vi "data analysis5.vi"() -> ()   [LabVIEW 2022 SP3]
uses:
  <vilib>/Utility/file.llb/Read From Spreadsheet File (DBL).vi
  <vilib>/Utility/file.llb/Read From Spreadsheet File (string).vi
  <vilib>/Utility/file.llb/Write To Spreadsheet File (DBL).vi
  <vilib>/Analysis/NI_AALBase.lvlib
panel:
  out "x+y 2":i32
  out "String converted to Time Stamp 2":timestamp
  out "output 2":timestamp
  out "Array":timestamp[](array[timestamp])
  out "Cursor.Cursor Position:Cursor X":dbl
  in  "Ring":u16(ring) items=["Temperature", "Humidity"]
  out "x+y":i32
  out "String converted to Time Stamp":timestamp
  out "Raw Data":dbl[][](graph)
  out "Time":string[](array[string])
  out "Temp":dbl[](array[numeric])
  out "Humid":dbl[](array[numeric])
  out "Current Data":dbl[](graph)
  in  "Log data value":bool
  out "standard deviation":dbl format="%0.2f"
  out "mean":dbl format="%0.2f"
  in  "stop":bool
  out "Data Section":dbl[][](graph)
  in  "Path":path=path "C:/Users/Deely/Desktop/test.txt"
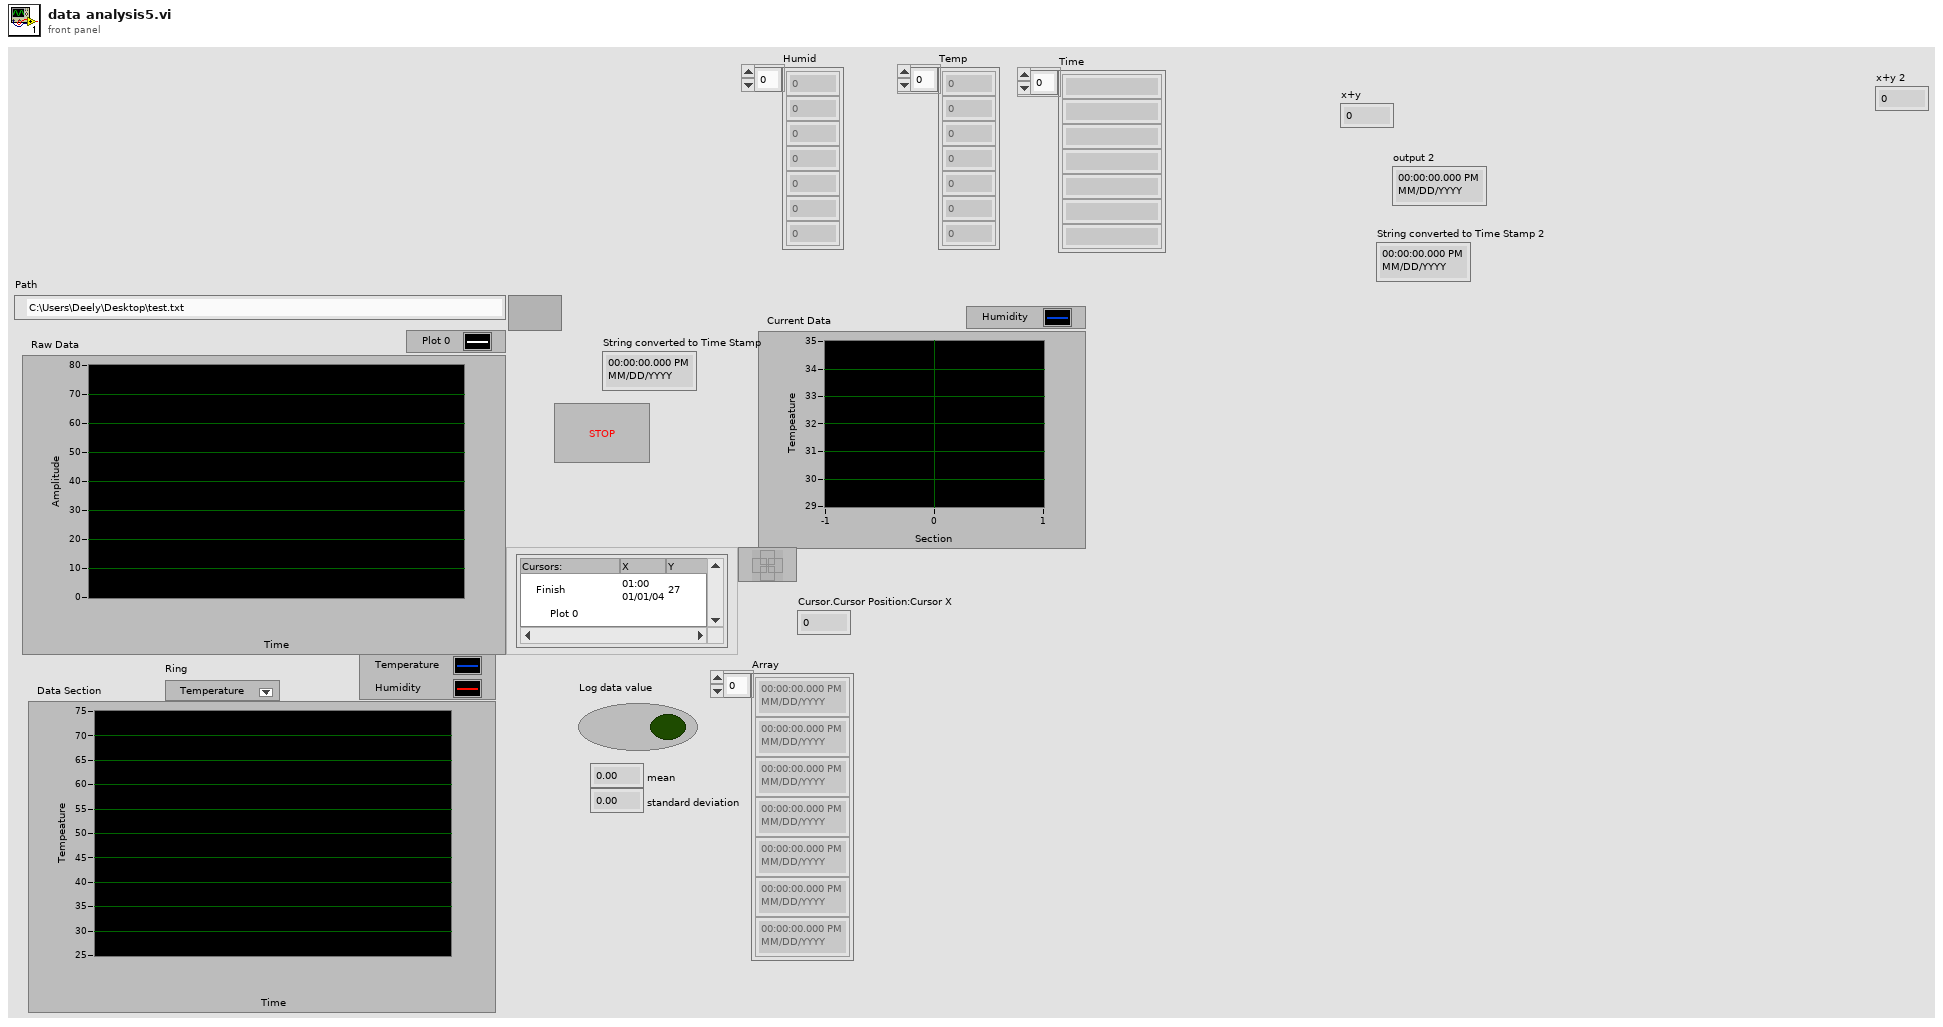
[diagram p1: front panel]
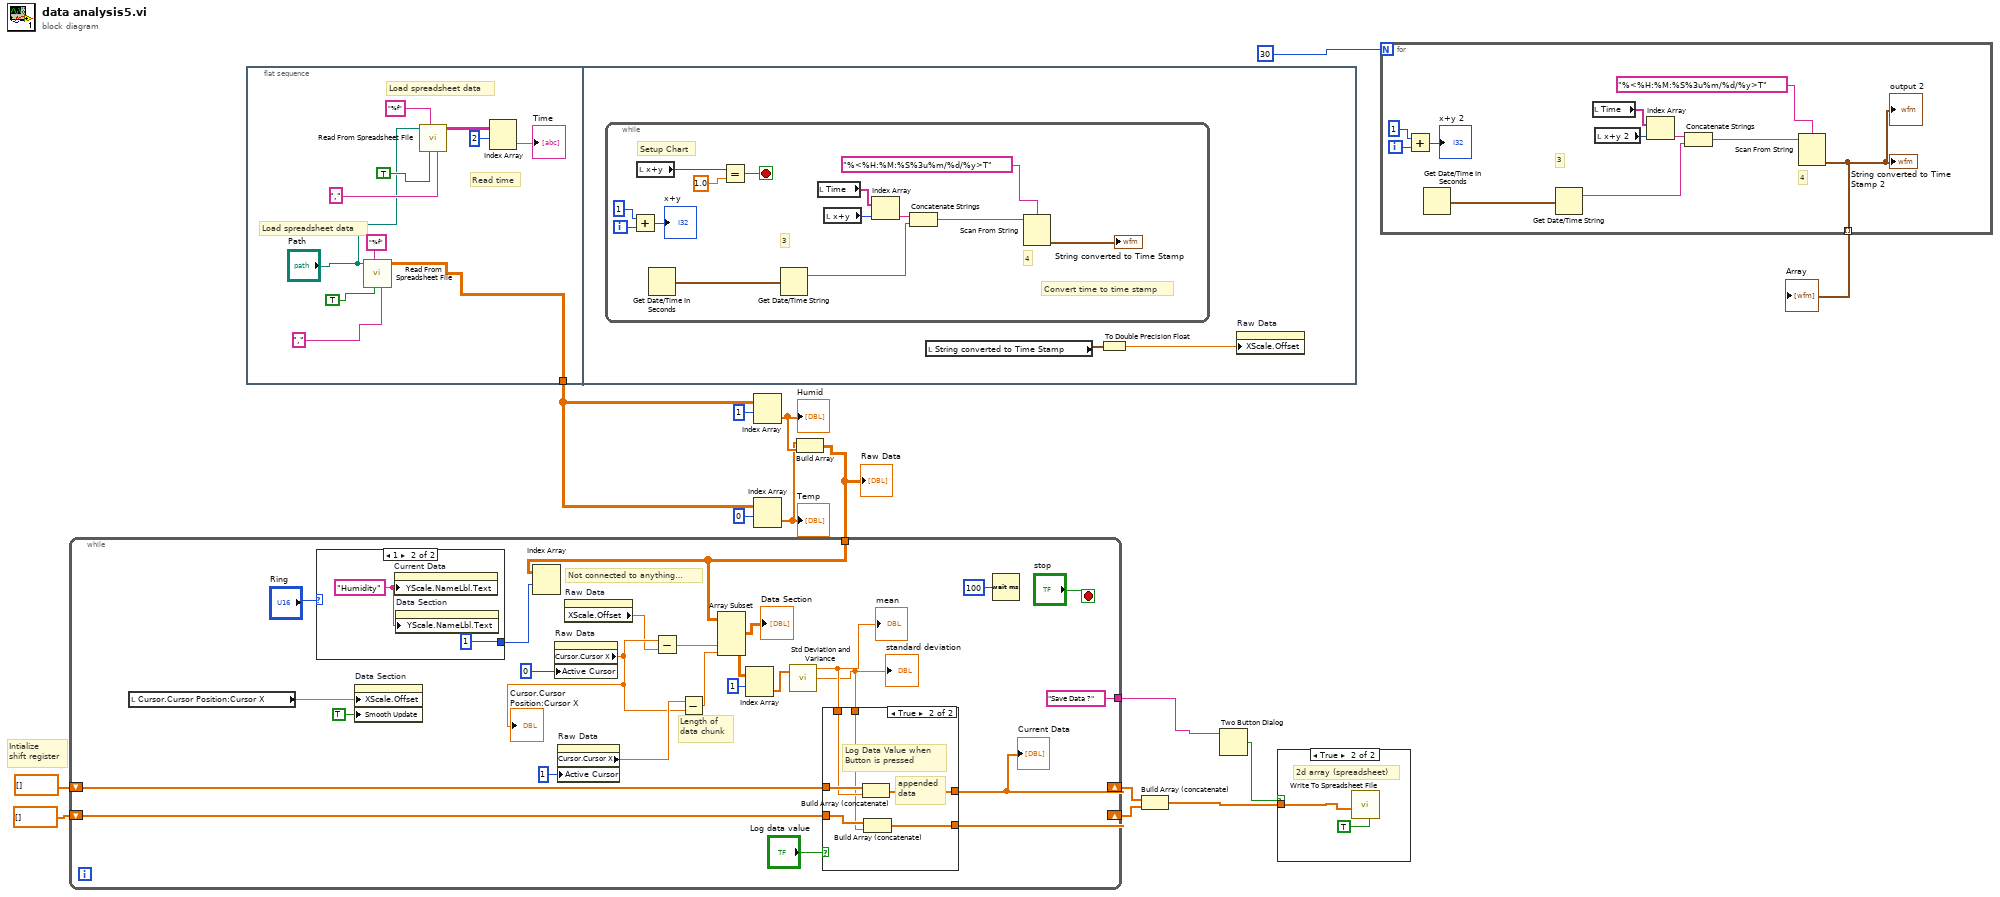
[diagram p0: block diagram]
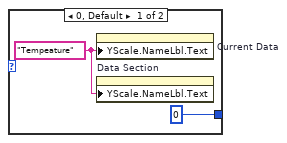
[diagram p3: hidden frame]
diagram:
  # "Intialize \nshift register"
  n1 = flat-sequence {
    tunnel: [w17] -> w1
    frame #0 {
      # "Read time"
      # "Load spreadsheet data"
      # "Load spreadsheet data"
      n2 = call-poly <vilib>:"Read From Spreadsheet File.vi"("delimiter (\\t)"=",", "transpose (no:F)"=TRUE, "format (%.3f)"="%f", "file path (dialog if empty)"="Path") -> ("all rows"=w17:dbl[][])  [unwired: 3 in, 4 out]
      n3 = call-poly <vilib>:"Read From Spreadsheet File.vi"("delimiter (\\t)"=",", "transpose (no:F)"=TRUE, "format (%s)"="%f" ("format (%.3f)"), "file path (dialog if empty)"="Path") -> ("all rows"=w19:string[][])  [unwired: 3 in, 4 out]
      n4 = Index Array(array=w19, index (row)=2) -> (element=→"Time":string[])  [unwired: 1 in]
    }
    frame #1 {
      n5 = while {
        i -> [w30]
        stop <- w31 stop-if-true
        # "Convert time to time stamp"
        # "4"
        # "3"
        # "Setup Chart"
        n6 = Add(x=1, y=w30) -> (x+y=→"x+y":i32)
        n7 = local read "x+y"() -> (w39:i32)
        n8 = Get Date/Time In Seconds() -> (seconds since 1Jan1904=w32:timestamp)
        n9 = Equal?(x=w39, y=1.0 ("x")) -> (x = y?=w31:bool)
        n10 = Get Date/Time String(seconds (now)=w32) -> (date string=w38:string)  [unwired: 3 out]
        n11 = local read "Time"() -> (w35:string[])
        n12 = local read "x+y"() -> (w34:i32)
        n13 = Index Array(array=w35, index=w34) -> (element=w33:string)
        n14 = Concatenate Strings "Concatenate Strings"(w33, w38) -> (w37:string)
        n15 = Scan From String "Scan From String"(format string="%<%H:%M:%S%3u%m/%d/%y>T" ("input string"), input string=w37) -> (output 1=→"String converted to Time Stamp":timestamp)  [unwired: 2 in, 4 out]
      }
      n16 = local read "String converted to Time Stamp"() -> (w28:timestamp)
      n17 = To Double Precision Float(number=w28) -> (double precision float=w27:dbl)
      n18 = property on="Raw Data" class="WFGraph (strict)"("XScale.Offset"=w27) -> ()  [unwired: 2 in, 2 out]
    }
  }
  n19 = Index Array(array=w1, index (row)=1) -> (element=w3:dbl[])  [unwired: 1 in]
  "Humid" <- w3
  n20 = Index Array(array=w1, index (row)=0) -> (element=w2:dbl[])  [unwired: 1 in]
  "Temp" <- w2
  n21 = Build Array(w2, w3) -> (w4:dbl[][])
  "Raw Data" <- w4
  n22 = while {
    shift-right: [w62] -> w12
    shift-left: dbl[] [] ("subarray") -> [w64]
    shift-right: [w59] -> w13
    shift-left: dbl[] [] ("subarray") -> [w61]
    tunnel: ["Save Data ?" ("message")] -> w9
    tunnel: w4 -> [w51]
    stop <- "stop" stop-if-true
    # "Not connected to anything…"
    # "Length of \ndata chunk"
    n23 = local read "Cursor.Cursor Position:Cursor X"() -> (w46:dbl)
    n24 = case shown="1" "Ring" {
      tunnel: [0 ("index (row)") 1 ("index (row)")] -> w54
      frame 0, Default {
        w68 = "Tempeature" ("Y Scale.Unit Label.Text")
        n25 = property on="Current Data" class="WFGraph (strict)"("YScale.NameLbl.Text"=w68) -> ()  [unwired: 2 in, 2 out]
        n26 = property on="Data Section" class="WFGraph (strict)"("YScale.NameLbl.Text"=w68) -> ()  [unwired: 2 in, 2 out]
      }
      frame 1 {
        w70 = "Humidity" ("Y Scale.Unit Label.Text")
        n27 = property on="Current Data" class="WFGraph (strict)"("YScale.NameLbl.Text"=w70) -> ()  [unwired: 2 in, 2 out]
        n28 = property on="Data Section" class="WFGraph (strict)"("YScale.NameLbl.Text"=w70) -> ()  [unwired: 2 in, 2 out]
      }
    }
    n29 = property on="Data Section" class="WFGraph (strict)"("XScale.Offset"=w46, "Smooth Update"=TRUE) -> ()  [unwired: 2 in, 2 out]
    n30 = Index Array(array=w51, index (row)=w54) -> ()  [unwired: 1 in, 1 out]
    n31 = property on="Raw Data" class="WFGraph (strict)"("Active Cursor"=u32 0) -> ("Cursor.Cursor X"=w45:dbl)  [unwired: 2 in, 2 out]
    "Cursor.Cursor Position:Cursor X" <- w45
    n32 = property on="Raw Data" class="WFGraph (strict)"("Active Cursor"=u32 1) -> ("Cursor.Cursor X"=w53:dbl)  [unwired: 2 in, 2 out]
    n33 = property on="Raw Data" class="WFGraph (strict)"() -> ("XScale.Offset"=w44:dbl)  [unwired: 2 in, 2 out]
    n34 = Subtract(x=w45, y=w44) -> (x-y=w43:dbl)
    n35 = Subtract(x=w53, y=w45) -> (x-y=w50:dbl)
    n36 = Array Subset(array=w51, index (col)=w43, length (col)=w50) -> (w49:dbl[][])  [unwired: 2 in]
    "Data Section" <- w49
    n37 = Index Array(array=w49, index (row)=1) -> (element=w48:dbl[])  [unwired: 1 in]
    n38 = call <vilib>:"Std Deviation and Variance.vi"("X"=w48) -> ("mean"=w63:dbl, "standard deviation"=w60:dbl)  [unwired: 1 in, 1 out]
    "mean" <- w63
    "standard deviation" <- w60
    n39 = case shown="True" "Log data value" {
      tunnel: w64 -> [w73 w79]
      tunnel: w63 -> [_ w78]
      tunnel: [w73 w77] -> w62
      tunnel: w61 -> [w72 w76]
      tunnel: w60 -> [_ w75]
      tunnel: [w72 w74] -> w59
      frame False {
        # "Do nothing just pass\n data through"
      }
      frame True {
        # "appended\ndata"
        # "Log Data Value when \nButton is pressed"
        n40 = Build Array (concatenate)(w79, w78) -> (w77:dbl[])
        n41 = Build Array (concatenate)(w76, w75) -> (w74:dbl[])
      }
    }
    "Current Data" <- w62
    n42 = Wait (ms)(milliseconds to wait=u32 100) -> ()  [unwired: 1 out]
  }
  n43 = Build Array (concatenate)(w12, w13) -> (w11:dbl[])
  n44 = Two Button Dialog(message=w9) -> (T button?=w10:bool)  [unwired: 2 in]
  n45 = case shown="True" w10 {
    tunnel: w11 -> [_ w81]
    frame False {
    }
    frame True {
      # "2d array (spreadsheet)"
      n46 = call-poly <vilib>:"Write To Spreadsheet File.vi"("transpose? (no:F)"=TRUE, "1D data"=w81) -> ()  [unwired: 6 in, 1 out]
    }
  }
  n47 = for {
    N: 30 -> [_]
    tunnel: [w82] -> w5 mode=indexing
    i -> [w83]
    # "4"
    # "3"
    n48 = Add(x=1, y=w83) -> (x+y=→"x+y 2":i32)
    n49 = Get Date/Time In Seconds() -> (seconds since 1Jan1904=w84:timestamp)
    n50 = Get Date/Time String(seconds (now)=w84) -> (date string=w90:string)  [unwired: 3 out]
    n51 = local read "Time"() -> (w87:string[])
    n52 = local read "x+y 2"() -> (w86:i32)
    n53 = Index Array(array=w87, index=w86) -> (element=w85:string)
    n54 = Concatenate Strings "Concatenate Strings"(w85, w90) -> (w89:string)
    n55 = Scan From String "Scan From String"(format string="%<%H:%M:%S%3u%m/%d/%y>T" ("input string"), input string=w89) -> (output 1=w82:timestamp)  [unwired: 2 in, 4 out]
    "String converted to Time Stamp 2" <- w82
    "output 2" <- w82
  }
  "Array" <- w5
